vi "Write Counter Driven State.vi"(8 "error in":errorcluster, 10 "counter driven state":T1, 11 "counter driven output channel in":refnum<class "Counter Driven Output Channel.lvclass">) -> (0 "error out":errorcluster, 3 "counter driven output channel out":refnum<class "Counter Driven Output Channel.lvclass">)   [LabVIEW 2017, in "Scan Engine Scripting.lvlib" / "Counter Driven Output Channel.lvclass"]
uses:
  Counter Driven Output Channel.lvclass
  Counter Driven State.ctl
  Counter Driven Output Channel.lvclass/Counter Driven Output Channel.ctl
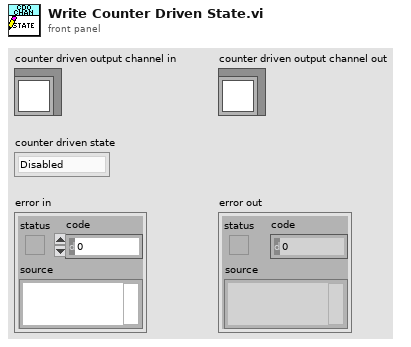
[diagram p1: front panel]
types:
  T1 = typedef "Scan Engine Scripting.lvlib/Counter Driven Output Channel.lvclass/Counter Driven State.ctl" = enum16{"Disabled", "Enabled"}
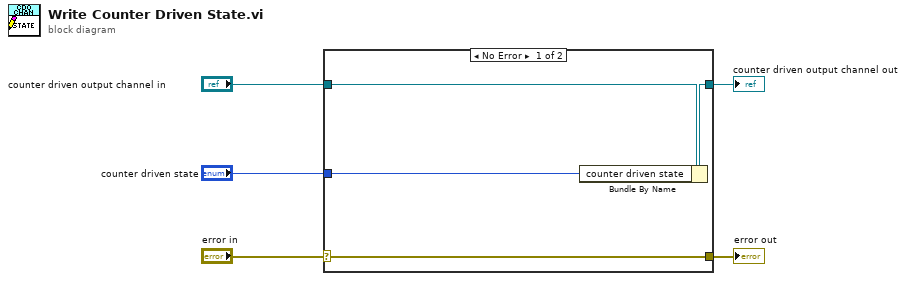
[diagram p0: block diagram]
diagram:
  n1 = case shown="No Error" "error in" {
    selector: "error in" -> [w9 w10]
    tunnel: [w9 w10] -> w4
    tunnel: [w7 w11] -> w2
    tunnel: "counter driven output channel in" -> [w8 w11]
    tunnel: "counter driven state" -> [w6 _]
    frame No Error {
      n2 = Bundle By Name(cluster=w8, "counter driven state"=w6) -> (w7:refnum<class "Counter Driven Output Channel.lvclass">)
    }
    frame Error {
    }
  }
  "error out" <- w4
  "counter driven output channel out" <- w2
